vi "Read Timing Override.vi"(8 "error in (no error)":errorcluster, 11 "CIFTemplateNode in":refnum<class "CIFCorePlugin.lvclass">) -> (0 "error out":errorcluster, 2 "Timing Overrides":T1, 3 "CIFTemplateNode out":refnum<class "CIFCorePlugin.lvclass">)   [LabVIEW 2021, in "CIFCorePlugin.lvclass"]
doc: "Set a timing override. Timing overrides allow programatic updates to change the timing behavior of the plugin. Skipping sleep is used when the plugin self times (normally for FIFO reads with timeout or driver reads for timing). The period will override the configuration of the plugin sleep timer."
uses:
  CIFCorePlugin.lvclass
  Common/Typedef/Timing Overrides.ctl
  CIFCorePlugin.lvclass/CIFCorePlugin.ctl
  Common/CIFCoreCommon.lvlib
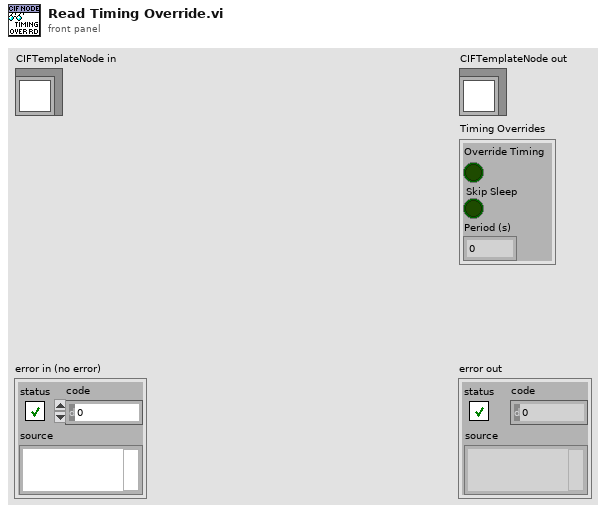
[diagram p1: front panel]
types:
  T1 = typedef "CIFCoreCommon.lvlib/Timing Overrides.ctl" = cluster{"Override Timing":bool, "Skip Sleep":bool, "Period (s)":dbl}
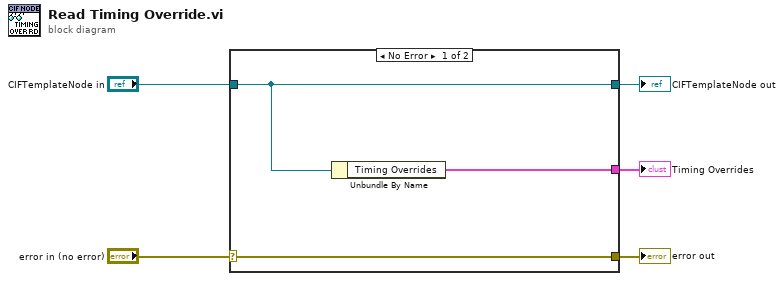
[diagram p0: block diagram]
diagram:
  n1 = case shown="No Error" "error in (no error)" {
    selector: "error in (no error)" -> [w8 w9]
    tunnel: [w8 w9] -> w4
    tunnel: [w7 w10] -> w2
    tunnel: "CIFTemplateNode in" -> [w7 w10]
    tunnel: [w6 _] -> w1
    frame No Error {
      n2 = Unbundle By Name(w7) -> ("Timing Overrides"=w6:T1)
    }
    frame Error {
    }
  }
  "error out" <- w4
  "CIFTemplateNode out" <- w2
  "Timing Overrides" <- w1
